vi "Set.vi"(10 "Point to Set":cluster{i64, i64, i64}, 11 "Internal?":bool) -> (3 "Set?":bool)   [LabVIEW 2021, in "d18.lvlib"]
uses:
  d18.lvlib
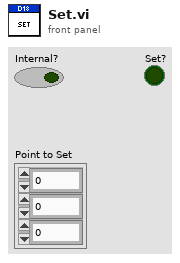
[diagram p1: front panel]
types:
  T1 = cluster{"Point to Set":cluster{i64, i64, i64}, "Internal?":bool}
  T2 = cluster{cluster{"Point to Set":cluster{i64, i64, i64}, "Internal?":bool}, "notifier out":refnum<notifier>}
  T3 = cluster{string, cluster{cluster{"Point to Set":cluster{i64, i64, i64}, "Internal?":bool}, "notifier out":refnum<notifier>}}
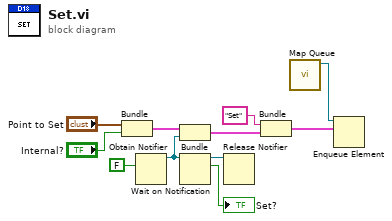
[diagram p0: block diagram]
diagram:
  n1 = Bundle("Point to Set"="Point to Set", "Internal?"="Internal?") -> (w3:T1)  [unwired: 1 in]
  n2 = Obtain Notifier(notification data type=FALSE ("Internal?")) -> (notifier out=w10:refnum<notifier>)  [unwired: 3 in, 2 out]
  n3 = Bundle(w3, "notifier out"=w10) -> (w9:T2)  [unwired: 1 in]
  n4 = Wait on Notification(notifier=w10) -> (notifier out=w11:refnum<notifier>, notification=→"Set?":bool)  [unwired: 3 in, 2 out]
  n5 = Release Notifier(notifier=w11) -> ()  [unwired: 2 in, 3 out]
  n6 = Bundle("Set", w9) -> (w7:T3)  [unwired: 1 in]
  n7 = call "Map Queue.vi"() -> ("Queue out"=w6:refnum<queue>)  [unwired: 11 in]
  n8 = Enqueue Element(queue=w6, element=w7) -> ()  [unwired: 2 in, 3 out]
